vi "MGCC_StaEst_funDSE.vi"() -> ()   [LabVIEW 2016]
panel:
  out "equ_c":dbl[](array[numeric])
  out "equ_d":dbl[](array[numeric])
  out "joc_c":dbl[][](array[numeric])
  out "joc_d":dbl[][](array[numeric])
  out "Ginv":dbl[][](array[numeric])
  out "G2":dbl[](array[numeric])
  out "equ_vn":dbl[](array[numeric])
  out "equ_pn":dbl[](array[numeric])
  out "equ_qn":dbl[](array[numeric])
  out "joc_vn":dbl[][](array[numeric])
  out "joc_pn":dbl[][](array[numeric])
  out "joc_qn":dbl[][](array[numeric])
  out "Loop number":i32
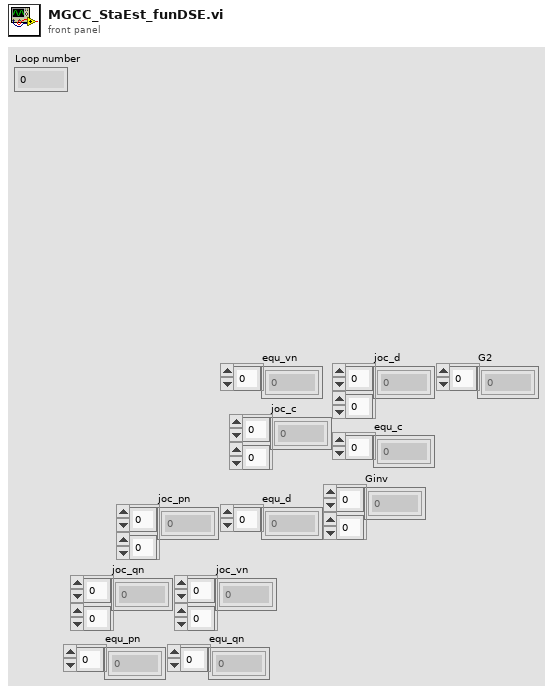
[diagram p1: front panel]
types:
  T1 = cluster{"Node":dbl, "Line":dbl, "StateVar":i32, "Zeroinj":i32}
  T2 = cluster{"PN":i32[][], "QN":i32[][], "VN":i32[][]}
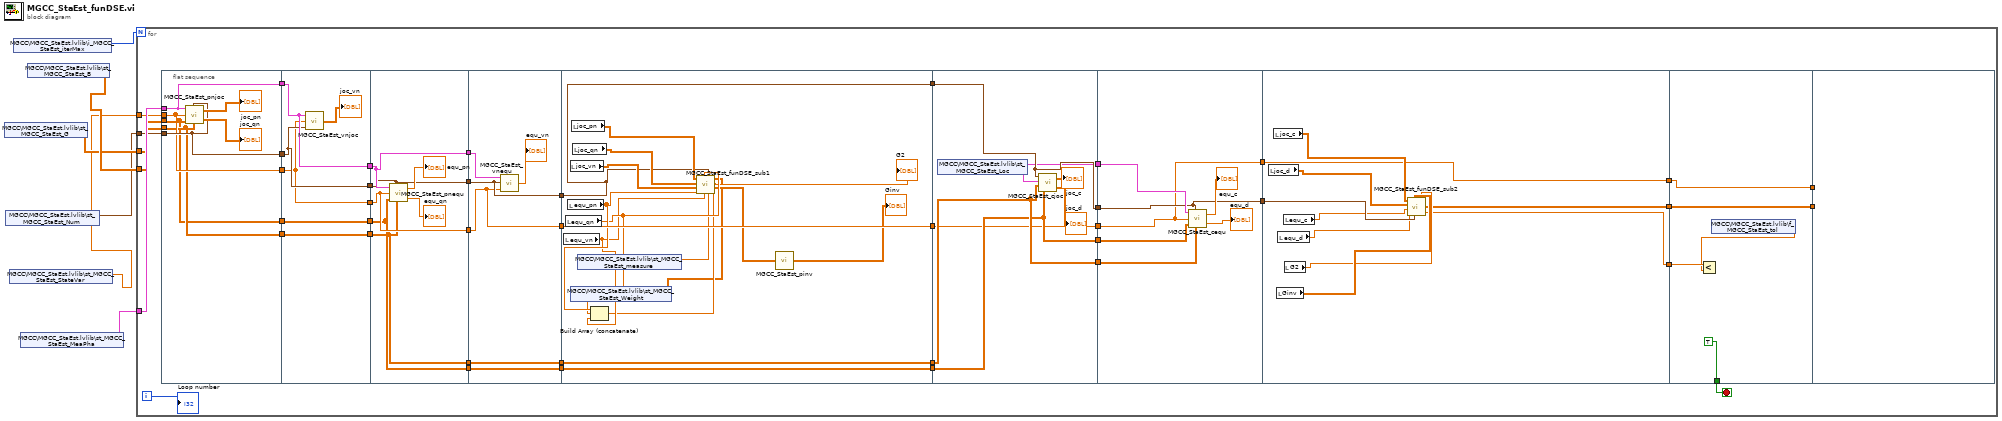
[diagram p0: block diagram]
diagram:
  n1 = shared-variable "MGCC\\MGCC_StaEst.lvlib\\st_MGCC_StaEst_G"() -> (w5:dbl[][])  [unwired: 1 in, 1 out]
  n2 = shared-variable "MGCC\\MGCC_StaEst.lvlib\\st_MGCC_StaEst_Num"() -> (w4:T1)  [unwired: 1 in, 1 out]
  n3 = shared-variable "MGCC\\MGCC_StaEst.lvlib\\st_MGCC_StaEst_StateVar"() -> (w1:dbl[])  [unwired: 1 in, 1 out]
  n4 = shared-variable "MGCC\\MGCC_StaEst.lvlib\\i_MGCC_StaEst_iterMax"() -> (w3:i32)  [unwired: 1 in, 1 out]
  n5 = shared-variable "MGCC\\MGCC_StaEst.lvlib\\st_MGCC_StaEst_MeaPha"() -> (w2:T2)  [unwired: 1 in, 1 out]
  n6 = shared-variable "MGCC\\MGCC_StaEst.lvlib\\st_MGCC_StaEst_B"() -> (w6:dbl[][])  [unwired: 1 in, 1 out]
  n7 = for {
    N: w3 -> [_]
    tunnel: w2 -> [w48]
    tunnel: w4 -> [w45]
    tunnel: w6 -> [w47]
    tunnel: w5 -> [w46]
    tunnel: w1 -> [w15]
    i -> [w13]
    stop <- w12 stop-if-true
    n8 = flat-sequence {
      tunnel: w48 -> [w53]
      tunnel: w47 -> [w49]
      tunnel: w46 -> [w50]
      tunnel: w45 -> [w52]
      tunnel: [w53] -> w44
      tunnel: [w52] -> w43
      tunnel: [w49] -> w38
      tunnel: [w50] -> w36
      tunnel: w15 -> [w51]
      tunnel: [w51] -> w14
      tunnel: w44 -> [w60]
      tunnel: w43 -> [w59]
      tunnel: [w60] -> w42
      tunnel: [w59] -> w41
      tunnel: [w56] -> w40
      tunnel: [w58] -> w39
      tunnel: w38 -> [w58]
      tunnel: [w57] -> w37
      tunnel: w36 -> [w57]
      tunnel: w14 -> [w56]
      tunnel: w42 -> [w66]
      tunnel: w41 -> [w65]
      tunnel: w40 -> [w64]
      tunnel: w39 -> [w62]
      tunnel: w37 -> [w63]
      tunnel: [w66] -> w35
      tunnel: [w65] -> w34
      tunnel: [w64] -> w33
      tunnel: [w63] -> w28
      tunnel: [w62] -> w25
      tunnel: w35 -> [w74]
      tunnel: w34 -> [w72]
      tunnel: w33 -> [w69]
      tunnel: [w72] -> w32
      tunnel: [w71] -> w29
      tunnel: w28 -> [w71]
      tunnel: [w70] -> w26
      tunnel: w25 -> [w70]
      tunnel: [w69] -> w18
      tunnel: w32 -> [w81]
      tunnel: [w81] -> w31
      tunnel: [w90] -> w30
      tunnel: w29 -> [w90]
      tunnel: [w89] -> w27
      tunnel: w26 -> [w89]
      tunnel: [w88] -> w19
      tunnel: w18 -> [w88]
      tunnel: w31 -> [w93]
      tunnel: w30 -> [w95]
      tunnel: w27 -> [w94]
      tunnel: [w91] -> w24
      tunnel: [w95] -> w23
      tunnel: [w94] -> w22
      tunnel: [w93] -> w21
      tunnel: [w92] -> w20
      tunnel: w19 -> [w92]
      tunnel: w24 -> [w104]
      tunnel: w23 -> [w102]
      tunnel: w22 -> [w103]
      tunnel: w21 -> [w99]
      tunnel: w20 -> [w98]
      tunnel: [w99] -> w17
      tunnel: [w98] -> w10
      tunnel: w17 -> [w112]
      tunnel: [w107] -> w16
      tunnel: [w106] -> w11
      tunnel: w10 -> [w106]
      tunnel: [w105] -> w7
      tunnel: w16 -> [w119]
      tunnel: [TRUE] -> w12
      tunnel: w11 -> [w117]
      tunnel: [w117] -> w9
      tunnel: [w116] -> w8
      tunnel: w7 -> [w116]
      tunnel: w9 -> [_]
      tunnel: w8 -> [_]
      frame #0 {
        n9 = call "MGCC_StaEst_pnjoc.vi"("MeaPha"=w53, "Num"=w52, "StateVar"=w51, "B"=w49, "G"=w50) -> ("joc_pn"=→"joc_pn":dbl[][], "joc_qn"=→"joc_qn":dbl[][])
      }
      frame #1 {
        n10 = call "MGCC_StaEst_vnjoc.vi"("Num"=w59, "StateVar"=w56, "MeaPha"=w60) -> ("joc_vn"=→"joc_vn":dbl[][])
      }
      frame #2 {
        n11 = call "MGCC_StaEst_pnequ.vi"("MeaPha"=w66, "Num"=w65, "StateVar"=w64, "B"=w62, "G"=w63) -> ("equ_pn"=→"equ_pn":dbl[], "equ_qn"=→"equ_qn":dbl[])
      }
      frame #3 {
        n12 = call "MGCC_StaEst_vnequ.vi"("StateVar"=w69, "Num"=w72, "MeaPha"=w74) -> ("equ_vn"=→"equ_vn":dbl[])
      }
      frame #4 {
        n13 = local read "equ_vn"() -> (w82:dbl[])
        n14 = local read "equ_qn"() -> (w83:dbl[])
        n15 = local read "equ_pn"() -> (w84:dbl[])
        n16 = local read "joc_vn"() -> (w85:dbl[][])
        n17 = shared-variable "MGCC\\MGCC_StaEst.lvlib\\st_MGCC_StaEst_Weight"() -> (w75:dbl[][])  [unwired: 1 in, 1 out]
        n18 = local read "joc_pn"() -> (w87:dbl[][])
        n19 = local read "joc_qn"() -> (w86:dbl[][])
        n20 = shared-variable "MGCC\\MGCC_StaEst.lvlib\\st_MGCC_StaEst_measure"() -> (w76:dbl[])  [unwired: 1 in, 1 out]
        n21 = Build Array (concatenate)(w84, w83, w82) -> (w80:dbl[])
        n22 = call "MGCC_StaEst_funDSE_sub1.vi"("MeaEqu"=w80, "Weight"=w75, "measure"=w76, "Num"=w81, "equ_vn"=w82, "equ_qn"=w83, "equ_pn"=w84, "joc_vn"=w85, "joc_qn"=w86, "joc_pn"=w87) -> ("G3"=w78:dbl[][], "G2"=→"G2":dbl[])
        n23 = call "MGCC_StaEst_pinv.vi"("G3"=w78) -> ("Ginv"=→"Ginv":dbl[][])
      }
      frame #5 {
        n24 = shared-variable "MGCC\\MGCC_StaEst.lvlib\\st_MGCC_StaEst_Loc"() -> (w91:cluster{"Zeroinj":i32[][], "Line":i32[][]})  [unwired: 1 in, 1 out]
        n25 = call "MGCC_StaEst_cjoc.vi"("B"=w94, "G"=w95, "Loc"=w91, "Num"=w93) -> ("joc_d"=→"joc_d":dbl[][], "joc_c"=→"joc_c":dbl[][])
      }
      frame #6 {
        n26 = call "MGCC_StaEst_cequ.vi"("Loc"=w104, "Num"=w99, "StateVar"=w98, "B"=w103, "G"=w102) -> ("equ_c"=→"equ_c":dbl[], "equ_d"=→"equ_d":dbl[])
      }
      frame #7 {
        n27 = local read "joc_d"() -> (w113:dbl[][])
        n28 = local read "joc_c"() -> (w114:dbl[][])
        n29 = local read "Ginv"() -> (w109:dbl[][])
        n30 = local read "equ_d"() -> (w110:dbl[])
        n31 = local read "equ_c"() -> (w111:dbl[])
        n32 = local read "G2"() -> (w108:dbl[])
        n33 = call "MGCC_StaEst_funDSE_sub2.vi"("joc_c"=w114, "Ginv"=w109, "joc_d"=w113, "equ_c"=w111, "Num"=w112, "equ_d"=w110, "G2"=w108) -> ("deltaX"=w105:dbl[][], "tol_temp"=w107:dbl[])
      }
      frame #8 {
        n34 = shared-variable "MGCC\\MGCC_StaEst.lvlib\\f_MGCC_StaEst_tol"() -> (w115:dbl)  [unwired: 1 in, 1 out]
        n35 = Less?(x=w119, y=w115) -> ()  [unwired: 1 out]
      }
      frame #9 {
      }
    }
    "Loop number" <- w13
  }
